vi "REACTOR_PARSE_SET_ALICATS.vi"(11 "String":string="ALICATS: aC1: 10.00 aC2: 20.00 aC3: 30.00 aC4: 40.00") -> (0 "CANAL4":dbl=20.0, 1 "CANAL3":dbl=25.0, 2 "CANAL2":dbl=20.0, 3 "CANAL1":dbl=25.0, 4 "ALICATS_SP":T1)   [LabVIEW 2017]
uses:
  SERIAL ALICATS/__s_SPali4.ctl
panel:
  out "subString":string
  # "ALICATS: aC1: 0.00 aC2: 0.00 aC3: 0.00 aC4: 0.00"
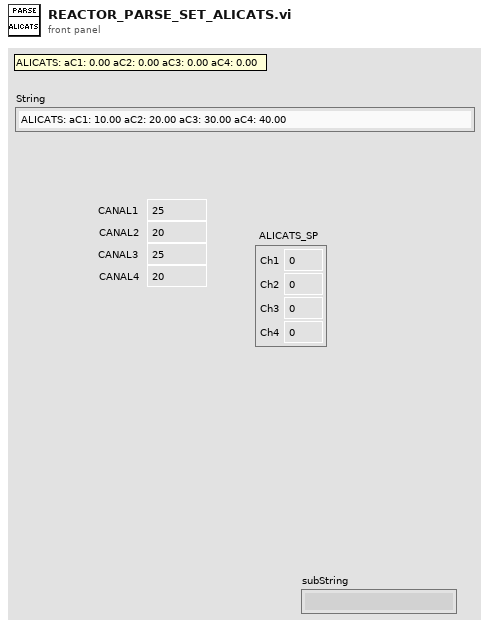
[diagram p1: front panel]
types:
  T1 = typedef "__s_SPali4.ctl" = cluster{"Ch1":dbl, "Ch2":dbl, "Ch3":dbl, "Ch4":dbl}
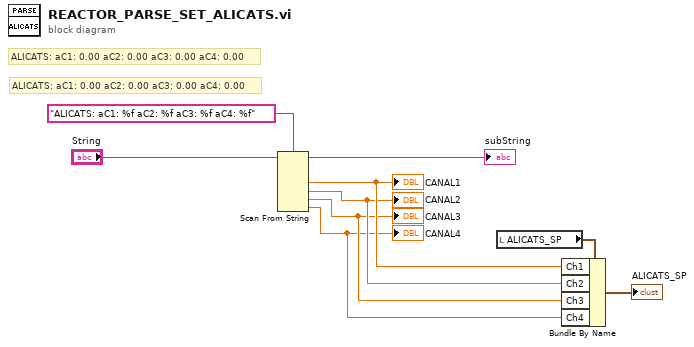
[diagram p0: block diagram]
diagram:
  # "ALICATS: aC1: 0.00 aC2: 0.00 aC3: 0.00 aC4: 0.00"
  # "ALICATS: aC1: 0.00 aC2: 0.00 aC3: 0.00 aC4: 0.00"
  n1 = Scan From String(format string="ALICATS: aC1: %f aC2: %f aC3: %f aC4: %f", input string="String") -> (remaining string=→"subString":string, output 1=w4:dbl, output 2=w3:dbl, output 3=w2:dbl, output 4=w1:dbl)  [unwired: 6 in, 2 out]
  "CANAL1" <- w4
  "CANAL2" <- w3
  "CANAL3" <- w2
  "CANAL4" <- w1
  n2 = local read "ALICATS_SP"() -> (w6:T1)
  n3 = Bundle By Name(cluster=w6, "Ch1"=w4, "Ch2"=w3, "Ch3"=w2, "Ch4"=w1) -> (→"ALICATS_SP":T1)
